vi "ReadnParse.vi"(11 "MAT Path":path) -> (0 "error out":errorcluster, 1 "Array":T2(array[cluster]), 2 "String out":string, 3 "Title":string)   [LabVIEW 2022 SP3]
uses:
  miDataType.ctl
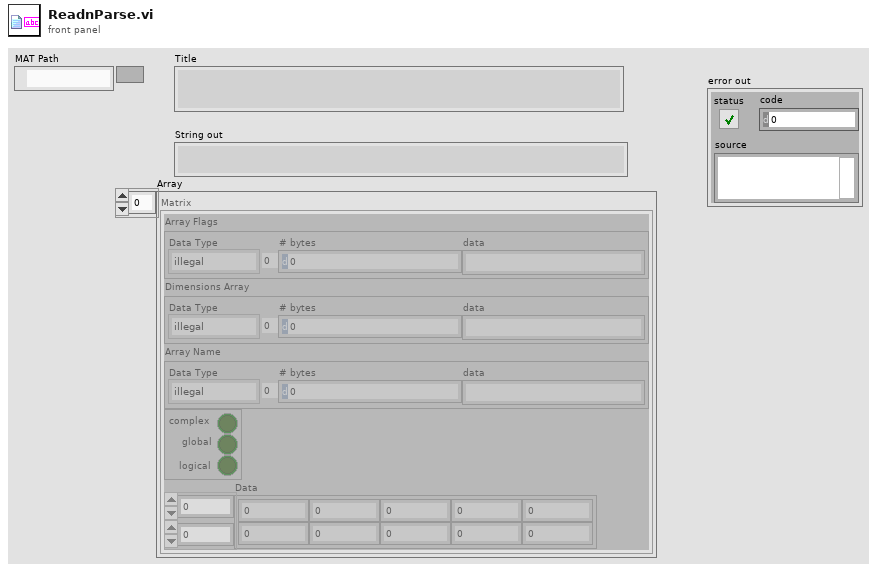
[diagram p1: front panel]
types:
  T1 = typedef "miDataType.ctl" = enum16{"illegal", "miINT8", "miUINT8", "miINT16", "miUINT16", "miINT32", "miUINT32", "miSINGLE", "--", "miDOUBLE", "---", "----", "miINT64", "miUINT64", "miMATRIX", "miCOMPRESSED", "miUTF8", "miUTF16", "miUTF32", "udefined"}
  T2 = cluster{"Array Flags":cluster{"Data Type":T1, "# bytes":u32, "data":string}, "Dimensions Array":cluster{"Data Type":T1, "# bytes":u32, "data":string}, "Array Name":cluster{"Data Type":T1, "# bytes":u32, "data":string}, cluster{"complex":bool, "global":bool, "logical":bool}, "Data":dbl[][]}[]
  T3 = enum16{"big-endian, network order", "native, host order", "little-endian"}
  T4 = cluster{"Data Type":T1, "# bytes":u32, "data":string}
  T5 = cluster{"Array Flags":cluster{"Data Type":T1, "# bytes":u32, "data":string}, "Dimensions Array":cluster{"Data Type":T1, "# bytes":u32, "data":string}, "Array Name":cluster{"Data Type":T1, "# bytes":u32, "data":string}, cluster{"complex":bool, "global":bool, "logical":bool}, "Data":dbl[][]}
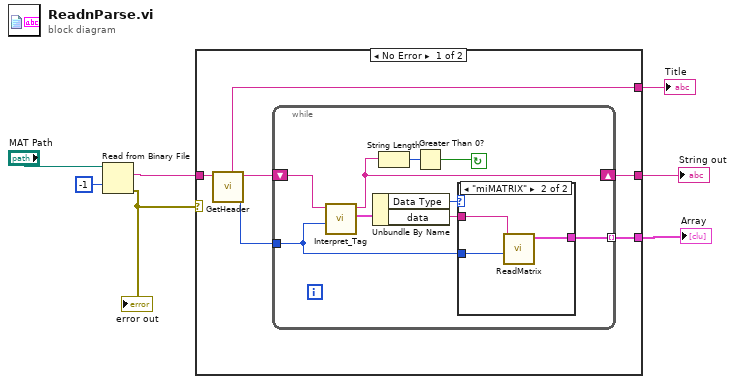
[diagram p0: block diagram]
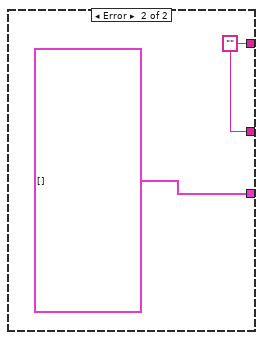
[diagram p3: hidden frame]
diagram:
  n1 = Read from Binary File(10:-1 ("count (1)"), 11:"MAT Path") -> (0:w1:errorcluster, 2:w3:string)  [unwired: 4 in, 2 out]
  "error out" <- w1
  n2 = case shown="No Error" w1 {
    tunnel: [w13 w27] -> w6
    tunnel: [w12 T2 []] -> w5
    tunnel: [w9 w27] -> w4
    tunnel: w3 -> [w8 _]
    frame No Error {
      n3 = call "GetHeader.vi"("String in"=w8) -> ("Endian"=w10:T3, "String out"=w11:string, "Title"=w9:string)  [unwired: 8 in]
      n4 = while {
        shift-right: [w16] -> w13
        shift-left: w11 -> [w21]
        tunnel: [w19] -> w12 mode=indexing
        tunnel: w10 -> [w18]
        stop <- w14 continue-if-true
        n5 = call "Interpret_Tag.vi"("byte order"=w18, "String in"=w21) -> ("Tag"=w22:T4, "String out"=w16:string)  [unwired: 7 in, 1 out]
        n6 = Unbundle By Name(w22) -> ("Data Type"=w17:T1, "data"=w20:string)
        n7 = String Length(string=w16) -> (length=w15:i32)
        n8 = Greater Than 0?(x=w15) -> (x > 0?=w14:bool)
        n9 = case shown="\"miMATRIX\"" w17 {
          tunnel: w20 -> [_ w25]
          tunnel: [_ w23] -> w19
          tunnel: w18 -> [_ w24]
          frame Default {
          }
          frame "miMATRIX" {
            n10 = call "ReadMatrix.vi"("byte order"=w24, "String in"=w25) -> ("Matrix"=w23:T5)  [unwired: 6 in, 3 out]
          }
        }
      }
    }
    frame Error {
      w27 = "" ("Title")
    }
  }
  "Title" <- w4
  "String out" <- w6
  "Array" <- w5
